vi "Apply_Parent_Settings.vi"(8 "error in (no error)":errorcluster, 10 "sourceItems in":refnum<class "AB_Source.lvclass">[](array[class]), 11 "AB_Source in":refnum<class "AB_Source.lvclass">) -> (0 "error out":errorcluster, 1 "parentApplies":T1, 2 "sourceItems out":refnum<class "AB_Source.lvclass">[](array[class]), 3 "AB_Source out":refnum<class "AB_Source.lvclass">)   [LabVIEW 2020, in "AB_Source.lvclass"]
uses:
  <vilib>/AppBuilder/AB_Classes/Source/AB_Source.lvclass
  <vilib>/AppBuilder/AB_Parent_Applies.ctl
  <vilib>/AppBuilder/AB_Classes/Source/AB_Source.lvclass/AB_Source.ctl
  <vilib>/AppBuilder/AB_Source_Property_Type.ctl
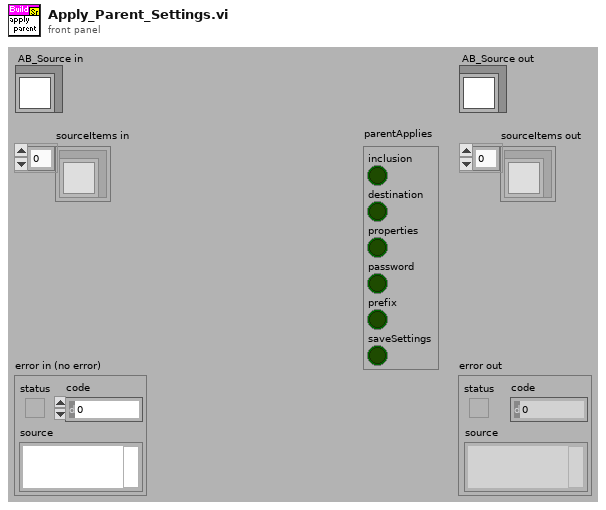
[diagram p1: front panel]
types:
  T1 = typedef "AB_Parent_Applies.ctl" = cluster{"inclusion":bool, "destination":bool, "properties":bool, "password":bool, "prefix":bool, "saveSettings":bool}
  T2 = typedef "AB_Source_Inclusion.ctl" = enum16{"IncludeIfReferenced", "Include", "Exclude", "TopLevel"}
  T3 = typedef "AB_Source_Properties.ctl" = cluster{"sourcePropertyType":T4, "value":variant}
  T4 = typedef "AB_Source_Property_Type.ctl" = enum16{"Remove block diagram", "Remove front panel", "Password", "Window has title bar", "Show menu bar", "Show vertical scroll bar", "Show horizontal scroll bar", "Show toolbar", "Show Abort button", "Show fp when called", "Window behavior", "Allow user to close window", "Window run-time position", "Run when opened", "Allow debugging", "Auto error handling", "Generate guard code", "Use stack variables", "Expression folding", "Integer only", "Inline subVI"}
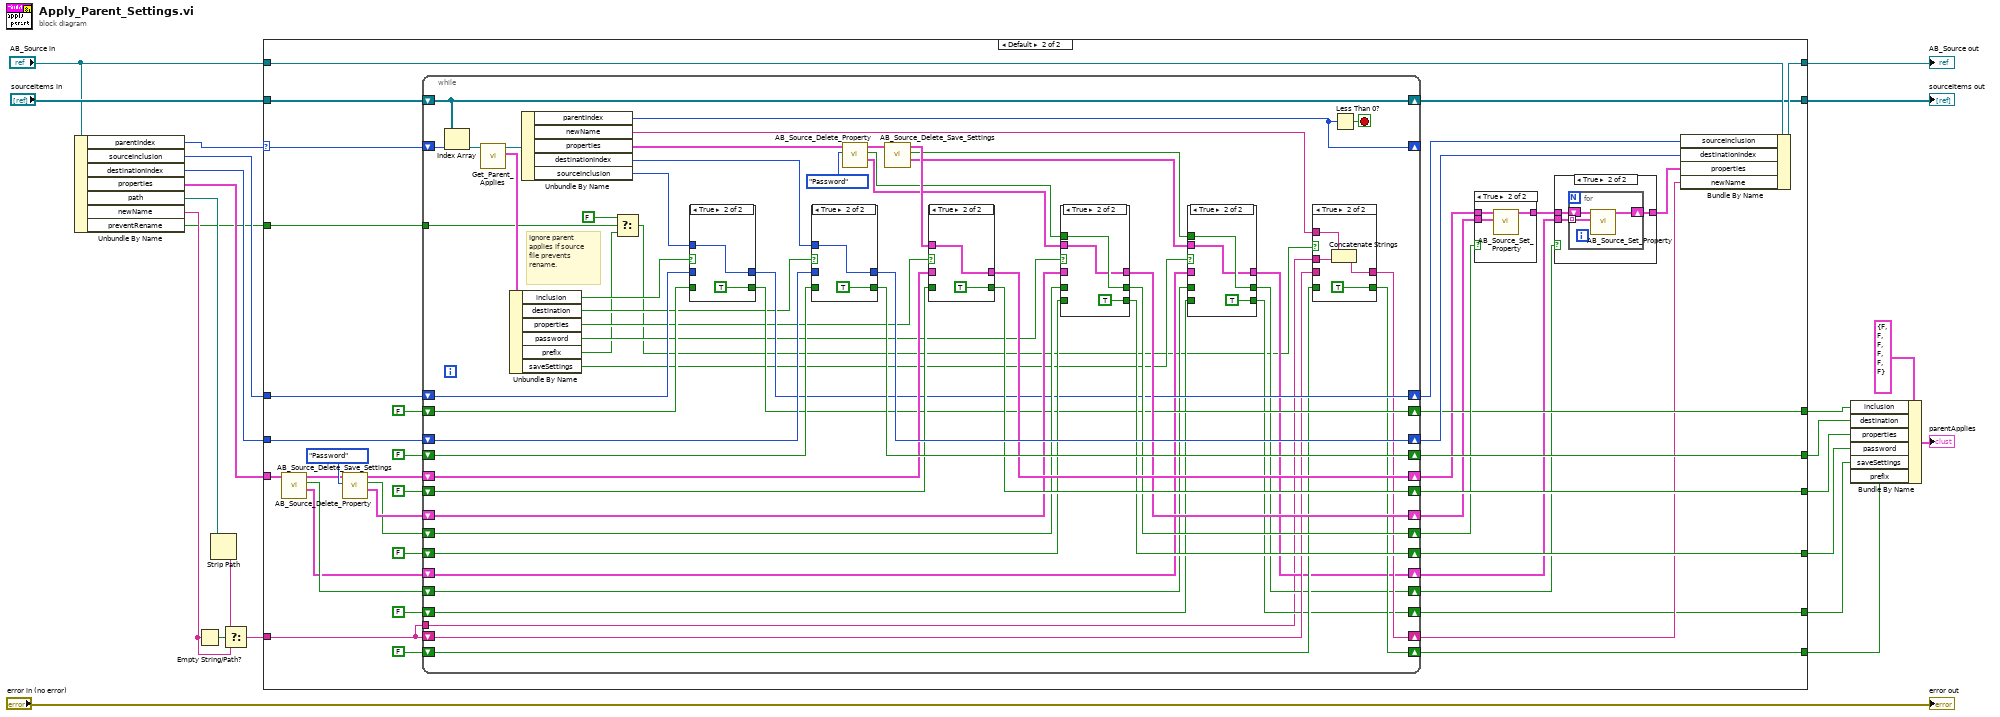
[diagram p0: block diagram]
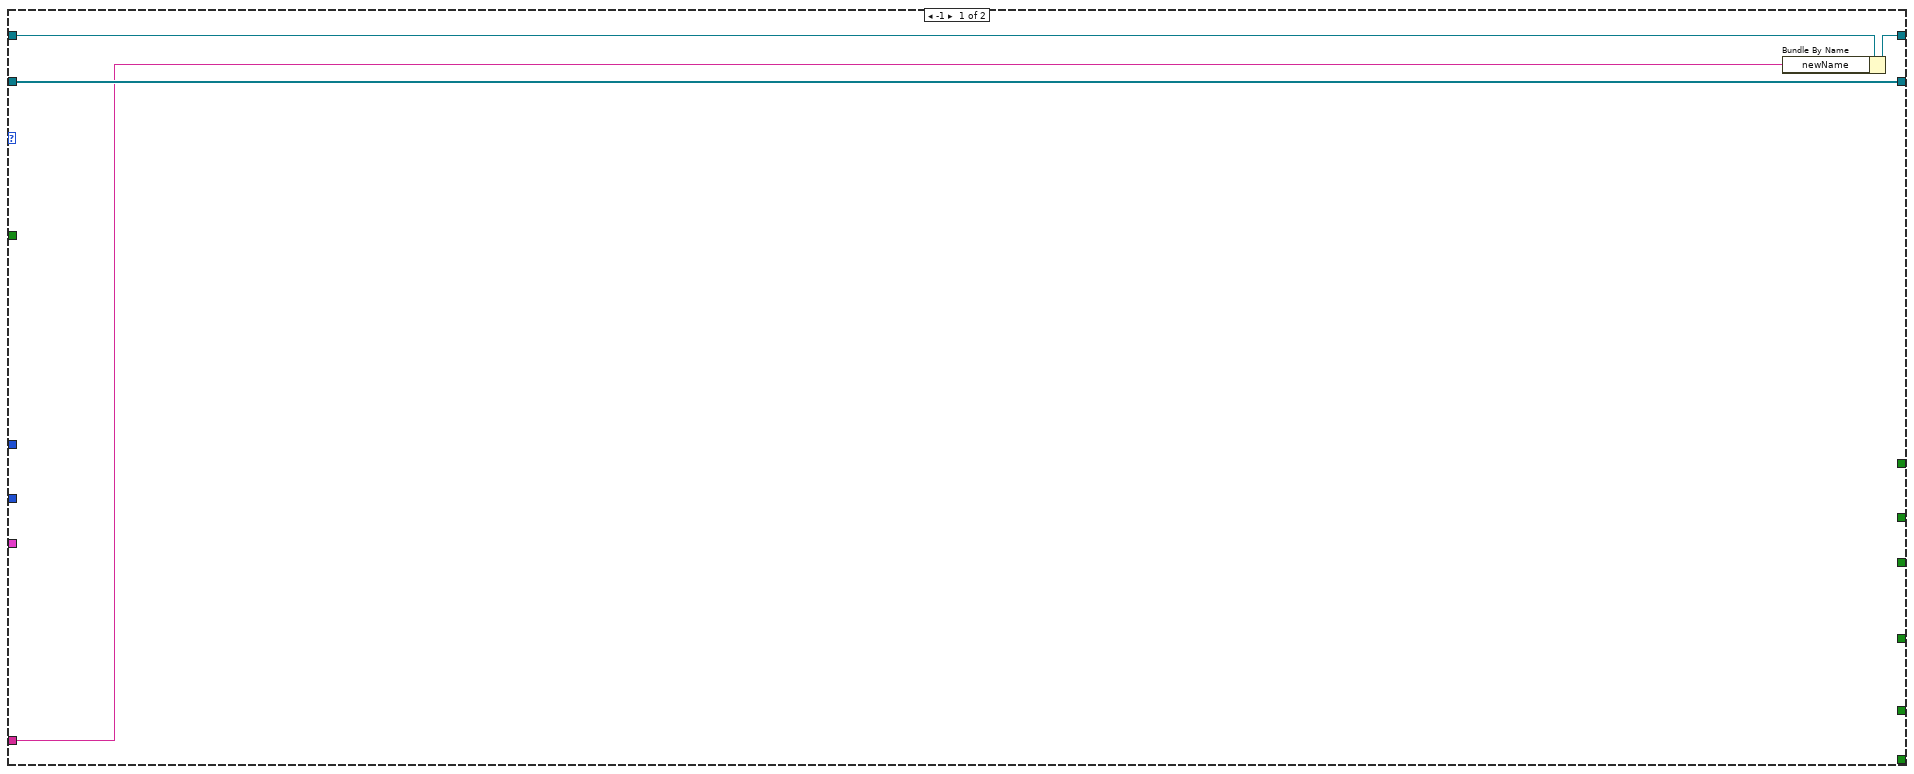
[diagram p2: hidden frame]
diagram:
  n1 = Unbundle By Name("AB_Source in") -> ("parentIndex"=w23:i32, "sourceInclusion"=w18:T2, "destinationIndex"=w20:i32, "properties"=w19:T3[], "path"=w4:path, "newName"=w7:string, "preventRename"=w1:bool)
  n2 = Empty String/Path?(string/path=w7) -> (empty?=w8:bool)
  n3 = Strip Path(path=w4) -> (name=w3:string)  [unwired: 1 out]
  n4 = Select(t=w3, s=w8, f=w7) -> (s? t:f=w6:string)
  n5 = case shown="Default" w23 {
    selector: w23 -> [_ w66]
    tunnel: [_ w64] -> w13
    tunnel: "sourceItems in" -> [w27 w63]
    tunnel: w20 -> [_ w62]
    tunnel: w19 -> [_ w38]
    tunnel: [_ w59] -> w12
    tunnel: [_ w58] -> w11
    tunnel: w18 -> [_ w56]
    tunnel: "AB_Source in" -> [w26 w55]
    tunnel: [w25 w52] -> w16
    tunnel: [_ w50] -> w14
    tunnel: [w27 w49] -> w15
    tunnel: w6 -> [w24 w29]
    tunnel: [_ w46] -> w5
    tunnel: [_ w34] -> w2
    tunnel: w1 -> [_ w28]
    frame -1 {
      n6 = Bundle By Name(cluster=w26, "newName"=w24) -> (w25:refnum<class "AB_Source.lvclass">)
    }
    frame Default {
      n7 = call <vilib>:"AB_Source_Delete_Save_Settings.vi"("sourceProperties in"=w38) -> ("saveSettings"=w35:T3[], "found"=w36:bool, "sourceProperties out"=w37:T3[])  [unwired: 1 in, 7 out]
      n8 = call <vilib>:"AB_Source_Delete_Property.vi"("type"=AB_Source_Property_Type."Password", "sourceProperties in"=w37) -> ("deletedProperty"=w43:T3, "found"=w42:bool, "sourceProperties out"=w45:T3[])  [unwired: 1 in, 6 out]
      n9 = while {
        shift-right: [w108] -> _
        shift-left: w66 -> [w133]
        shift-right: [w128] -> w64
        shift-left: FALSE -> [w127]
        shift-right: [w131] -> w49
        shift-left: w63 -> [w131]
        shift-right: [w130] -> w53
        shift-left: w62 -> [w129]
        shift-right: [w121] -> w40
        shift-left: w43 -> [w122]
        shift-right: [w117] -> w51
        shift-left: w42 -> [w120]
        shift-right: [w123] -> w59
        shift-left: FALSE -> [w125]
        shift-right: [w124] -> w41
        shift-left: w45 -> [w126]
        shift-right: [w118] -> w58
        shift-left: FALSE -> [w119]
        shift-right: [w114] -> w50
        shift-left: FALSE -> [w115]
        shift-right: [w113] -> w54
        shift-left: w56 -> [w116]
        shift-right: [w112] -> w46
        shift-left: FALSE -> [w109]
        shift-right: [w111] -> w47
        shift-left: w29 -> [w110]
        shift-right: [w95] -> w30
        shift-left: w35 -> [w98]
        shift-right: [w94] -> w31
        shift-left: w36 -> [w97]
        shift-right: [w93] -> w34
        shift-left: FALSE -> [w96]
        tunnel: w29 -> [w83]
        tunnel: w28 -> [w82]
        stop <- w132 stop-if-true
        # "Ignore parent applies if source file prevents rename."
        n10 = Index Array(array=w131, index=w133) -> (element=w86:refnum<class "AB_Source.lvclass">)
        n11 = call-dynamic "Get_Parent_Applies.vi"("AB_Source in"=w86) -> ("parentApplies"=w84:T1, "AB_Source out"=w85:refnum<class "AB_Source.lvclass">)  [unwired: 1 in, 8 out]
        n12 = Unbundle By Name(w84) -> ("inclusion"=w107:bool, "destination"=w106:bool, "properties"=w105:bool, "password"=w104:bool, "prefix"=w79:bool, "saveSettings"=w80:bool)
        n13 = Unbundle By Name(w85) -> ("parentIndex"=w108:i32, "newName"=w103:string, "properties"=w101:T3[], "destinationIndex"=w100:i32, "sourceInclusion"=w99:T2)
        n14 = Select(t=FALSE, s=w82, f=w79) -> (s? t:f=w78:bool)
        n15 = case shown="True" w107 {
          tunnel: [w147 w148] -> w113
          tunnel: w116 -> [w147 _]
          tunnel: [w146 TRUE] -> w114
          tunnel: w115 -> [w146 _]
          tunnel: w99 -> [_ w148]
          frame False {
          }
          frame True {
          }
        }
        n16 = case shown="True" w106 {
          tunnel: [w161 w162] -> w130
          tunnel: w129 -> [w161 _]
          tunnel: [w160 TRUE] -> w128
          tunnel: w127 -> [w160 _]
          tunnel: w100 -> [_ w162]
          frame False {
          }
          frame True {
          }
        }
        n17 = call <vilib>:"AB_Source_Delete_Property.vi"("type"=AB_Source_Property_Type."Password", "sourceProperties in"=w101) -> ("deletedProperty"=w89:T3, "found"=w90:bool, "sourceProperties out"=w92:T3[])  [unwired: 1 in, 6 out]
        n18 = call <vilib>:"AB_Source_Delete_Save_Settings.vi"("sourceProperties in"=w92) -> ("saveSettings"=w87:T3[], "found"=w88:bool, "sourceProperties out"=w91:T3[])  [unwired: 1 in, 7 out]
        n19 = case shown="True" w105 {
          tunnel: [w157 w158] -> w124
          tunnel: w126 -> [w157 _]
          tunnel: [w156 TRUE] -> w123
          tunnel: w125 -> [w156 _]
          tunnel: w91 -> [_ w158]
          frame False {
          }
          frame True {
          }
        }
        n20 = case shown="True" w104 {
          tunnel: [w152 w153] -> w121
          tunnel: w122 -> [w152 _]
          tunnel: [w151 w154] -> w117
          tunnel: w120 -> [w151 _]
          tunnel: w89 -> [_ w153]
          tunnel: [w150 TRUE] -> w118
          tunnel: w119 -> [w150 _]
          tunnel: w90 -> [_ w154]
          frame False {
          }
          frame True {
          }
        }
        n21 = case shown="True" w80 {
          tunnel: [w136 w137] -> w95
          tunnel: w98 -> [w136 _]
          tunnel: [w135 w138] -> w94
          tunnel: w97 -> [w135 _]
          tunnel: w87 -> [_ w137]
          tunnel: [w134 TRUE] -> w93
          tunnel: w96 -> [w134 _]
          tunnel: w88 -> [_ w138]
          frame False {
          }
          frame True {
          }
        }
        n22 = case shown="True" w78 {
          tunnel: [w141 w144] -> w111
          tunnel: w110 -> [w141 _]
          tunnel: [w140 TRUE] -> w112
          tunnel: w109 -> [w140 _]
          tunnel: w103 -> [_ w143]
          tunnel: w83 -> [_ w142]
          frame False {
          }
          frame True {
            n23 = Concatenate Strings(w143, w142) -> (w144:string)
          }
        }
        n24 = Less Than 0?(x=w108) -> (x < 0?=w132:bool)
      }
      n25 = case shown="True" w51 {
        tunnel: w41 -> [w74 w77]
        tunnel: [w74 w76] -> w33
        tunnel: w40 -> [_ w75]
        frame False {
        }
        frame True {
          n26 = call <vilib>:"AB_Source_Set_Property.vi"("sourceProperty"=w75, "sourceProperties in"=w77) -> ("sourceProperties out"=w76:T3[])  [unwired: 1 in, 8 out]
        }
      }
      n27 = case shown="True" w31 {
        tunnel: w33 -> [w67 w70]
        tunnel: [w67 w69] -> w32
        tunnel: w30 -> [_ w68]
        frame False {
        }
        frame True {
          n28 = for {
            shift-right: [w72] -> w69
            shift-left: w70 -> [w73]
            tunnel: w68 -> [w71] mode=indexing
            n29 = call <vilib>:"AB_Source_Set_Property.vi"("sourceProperty"=w71, "sourceProperties in"=w73) -> ("sourceProperties out"=w72:T3[])  [unwired: 1 in, 8 out]
          }
        }
      }
      n30 = Bundle By Name(cluster=w55, "sourceInclusion"=w54, "destinationIndex"=w53, "properties"=w32, "newName"=w47) -> (w52:refnum<class "AB_Source.lvclass">)
    }
  }
  "AB_Source out" <- w16
  "sourceItems out" <- w15
  n31 = Bundle By Name(cluster=T1 {"inclusion"=FALSE, "destination"=FALSE, "properties"=FALSE, "password"=FALSE, "prefix"=FALSE, "saveSettings"=FALSE} ("containerApplies"), "inclusion"=w14, "destination"=w13, "properties"=w12, "password"=w11, "saveSettings"=w2, "prefix"=w5) -> (→"parentApplies":T1)
  "error out" <- "error in (no error)"
